vi "Get Change.vi"(8 "error in (no error)":errorcluster, 10 "Cambio":dbl, 11 "User Interface in":refnum<class "User Interface.lvclass">) -> (0 "error out":errorcluster, 3 "User Interface out":refnum<class "User Interface.lvclass">)   [LabVIEW 2021, in "User Interface.lvlib" / "User Interface.lvclass"]
uses:
  User Interface.lvclass
  User Interface.lvclass/User Interface.ctl
  Dinero Messages/Change update Msg/Change update Msg.lvclass/Change update Msg.ctl
  <vilib>/ActorFramework/Message Enqueuer/Message Enqueuer.lvclass/Message Enqueuer.ctl
  <vilib>/ActorFramework/Message Enqueuer/Enqueue.vi
  Dinero Messages/Change update Msg/Change update Msg.lvclass
  C:/Program Files (x86)/National Instruments/LabVIEW 2021/vi.lib/ActorFramework/Message/Message.lvclass
  <vilib>/ActorFramework/Message Priority Queue/Priority Enqueue.vi
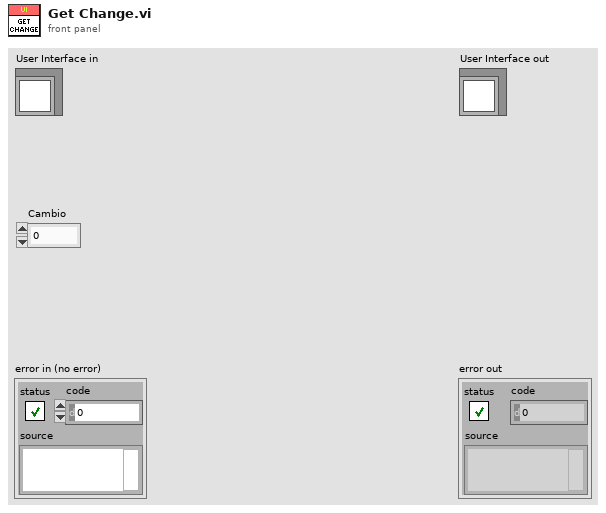
[diagram p1: front panel]
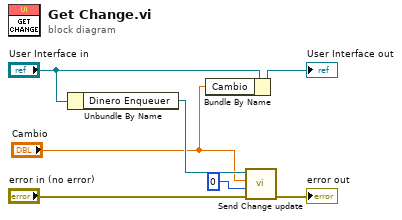
[diagram p0: block diagram]
diagram:
  n1 = Unbundle By Name("User Interface in") -> ("Dinero Enqueuer"=w3:refnum<class "Message Enqueuer.lvclass">)
  n2 = Bundle By Name(cluster="User Interface in", "Cambio"="Cambio") -> (→"User Interface out":refnum<class "User Interface.lvclass">)
  n3 = call "Send Change update.vi"("error in (no error)"="error in (no error)", "Credit"=0 ("Credito"), "Change"="Cambio", "Message Enqueuer"=w3) -> ("error out"=→"error out":errorcluster)  [unwired: 6 in, 1 out]
